vi "VSS Detection Frame Enemy.vi"(8 "error in":errorcluster, 9 "Array":u8[](array[numeric]) format="%02x") -> (0 "error out":errorcluster, 3 "Detection Frame":T1 {"robots_blue"."orientation" format="%+4.3f"; "robots_blue"."y" format="%+4.3f"; "robots_blue"."confidence" format="%4.3f"; "robots_blue"."x" format="%+4.3f"; "robots_yellow"."orientation" format="%+4.3f"; "robots_yellow"."y" format="%+4.3f"; "robots_yellow"."confidence" format="%4.3f"; "robots_yellow"."x" format="%+4.3f"})   [LabVIEW 2017]
uses:
  SSL Detection Frame.ctl
  SSL Detection Robot.ctl
  <vilib>/Analysis/Matrix/Datatypes/RealMatrix.ctl
  SSL Detection Ball.ctl
  <vilib>/Analysis/Matrix/NI_Matrix.lvlib
panel:
  out "size(s) 3":i32
  out "array w/ subset deleted out":u8[](array[numeric])
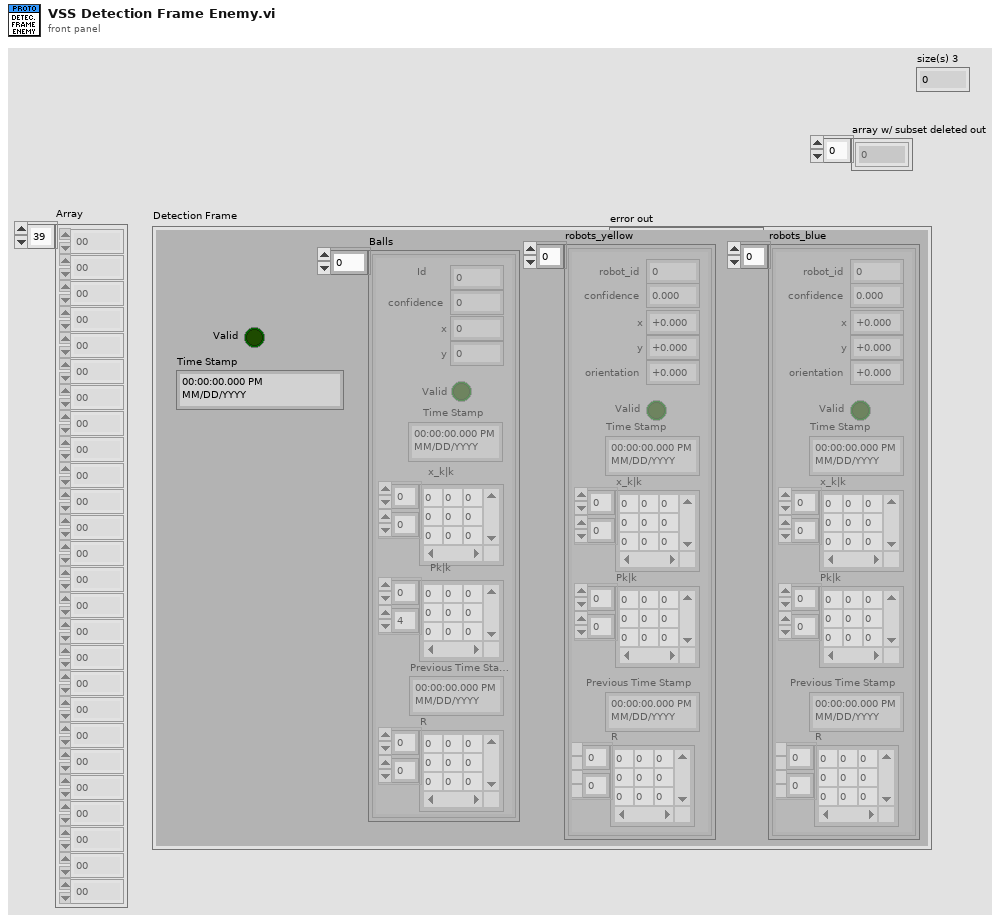
[diagram p1: front panel]
types:
  T1 = typedef "SSL Detection Frame.ctl" = cluster{"robots_yellow":T2[], "robots_blue":T2[], "Valid":bool, "Time Stamp":timestamp, "Balls":T4[]}
  T2 = typedef "SSL Detection Robot.ctl" = cluster{"x":sgl, "robot_id":u32, "confidence":sgl, "y":sgl, "orientation":sgl, "Valid":bool, "Time Stamp":timestamp, "x_k|k":T3, "Pk|k":T3, "Previous Time Stamp":timestamp, "R":T3}
  T3 = typedef "NI_Matrix.lvlib/RealMatrix.ctl" = dbl[][]
  T4 = typedef "SSL Detection Ball.ctl" = cluster{"x":sgl, "confidence":sgl, "y":sgl, "Valid":bool, "Time Stamp":timestamp, "x_k|k":T3, "Pk|k":T3, "Id":u32, "Previous Time Stamp":timestamp, "R":T3}
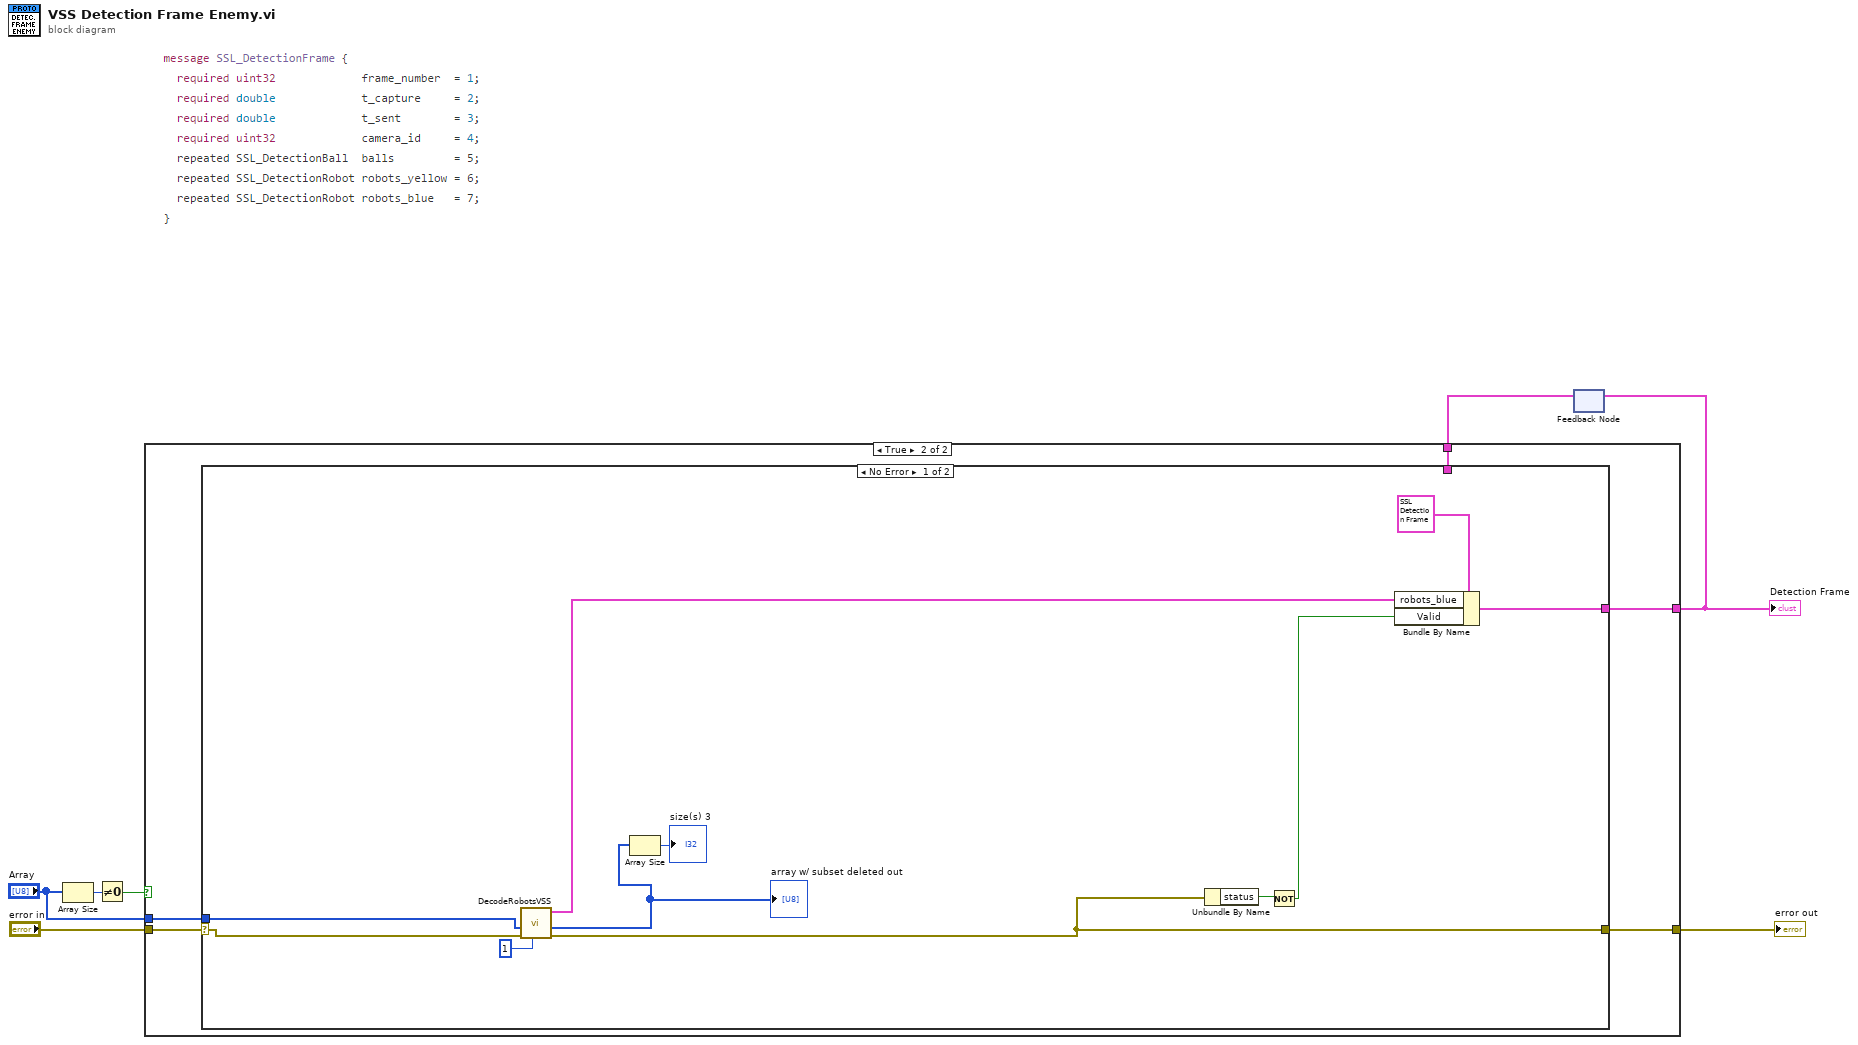
[diagram p0: block diagram]
diagram:
  n1 = Array Size(array="Array") -> (size(s)=w5:i32)
  n2 = Not Equal To 0?(x=w5) -> (x != 0?=w3:bool)
  n3 = feedback #1() -> (w2:T1)  [unwired: 1 in]
  n4 = case shown="True" w3 {
    tunnel: "error in" -> [_ w13]
    tunnel: "Array" -> [_ w12]
    tunnel: [_ w11] -> w4
    tunnel: [w8 w10] -> w1
    tunnel: w2 -> [w8 w9]
    frame False {
    }
    frame True {
      n5 = case shown="No Error" w13 {
        selector: w13 -> [w15 w26]
        tunnel: [w19 w26] -> w11
        tunnel: w12 -> [w14 _]
        tunnel: [w22 w25] -> w10
        tunnel: w9 -> [_ w25]
        frame No Error {
          n6 = call "DecodeRobotsVSS.vi"("offset"=1, "error in (no error)"=w15, "array w/ subset deleted in"=w14) -> ("error out"=w19:errorcluster, "array w/ subset deleted out"=w18:u8[], "Array"=w21:T2[])  [unwired: 5 in]
          "array w/ subset deleted out" <- w18
          n7 = Array Size(array=w18) -> (size(s)=→"size(s) 3":i32)
          n8 = Unbundle By Name(w19) -> ("status"=w20:bool)
          n9 = Not(x=w20) -> (.not. x?=w23:bool)
          n10 = Bundle By Name(cluster=T1 {"robots_yellow"=[], "robots_blue"=[], "Valid"=FALSE, "Time Stamp"=timestamp(0 s since 1904-01-01), "Balls"=[]} ("Detection Frame 2"), "robots_blue"=w21, "Valid"=w23) -> (w22:T1)
        }
        frame Error {
        }
      }
    }
  }
  "error out" <- w4
  "Detection Frame" <- w1
  n11 = feedback-in #1(w1) -> ()
